vi "CylNumand720Signal.vi"(11 "CurrentCAD":fxp<+,18,11> format="%.11g") -> (2 "数值输入控件":u8)   [LabVIEW 2020]
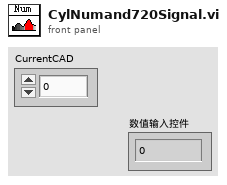
[diagram p1: front panel]
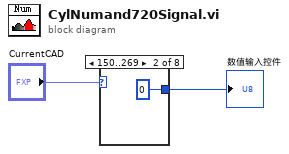
[diagram p0: block diagram]
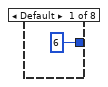
[diagram p2: hidden frame]
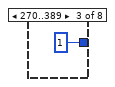
[diagram p3: hidden frame]
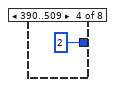
[diagram p4: hidden frame]
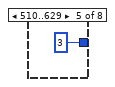
[diagram p5: hidden frame]
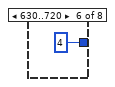
[diagram p6: hidden frame]
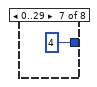
[diagram p7: hidden frame]
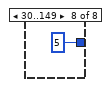
[diagram p8: hidden frame]
diagram:
  n1 = case shown="150..269" "CurrentCAD" {
    tunnel: [u8 6 u8 0 u8 1 u8 2 u8 3 u8 4 u8 4 u8 5] -> w1
    frame Default {
    }
    frame 150..269 {
    }
    frame 270..389 {
    }
    frame 390..509 {
    }
    frame 510..629 {
    }
    frame 630..720 {
    }
    frame 0..29 {
    }
    frame 30..149 {
    }
  }
  "数值输入控件" <- w1
